vi "Start Power Meter Sweep.vi"(8 "error in (no error)":errorcluster, 10 "Power Meter Sweep (1: Pause)":i32(ring)=1 items=["Run", "Pause"], 11 "VISA resource name":refnum<visa-resource-name>) -> (0 "error out":errorcluster, 3 "VISA resource name out":refnum<visa-resource-name>)   [LabVIEW 2022 SP3, in "Agilent N934X Series.lvlib"]
doc: "Enables or disables power meter sweep state.\n\nNote:\nThis VI is only applicable for N9321C, N9322C, N9323C, N9324C."
uses:
  <instrlib>/Agilent N934X Series/Agilent N934X Series.lvlib
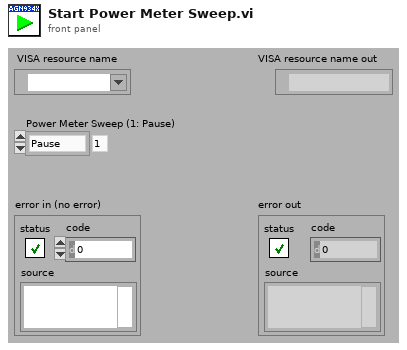
[diagram p1: front panel]
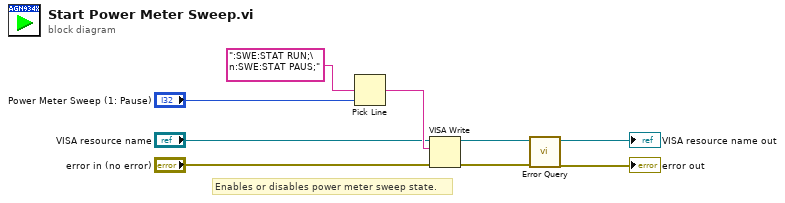
[diagram p0: block diagram]
diagram:
  # "Enables or disables power meter sweep state."
  n1 = Pick Line(multi-line string=":SWE:STAT RUN;\n:SWE:STAT PAUS;", line index="Power Meter Sweep (1: Pause)") -> (output string=w7:string)  [unwired: 1 in]
  n2 = VISA Write(VISA resource name="VISA resource name", write buffer=w7, error in (no error)="error in (no error)") -> (VISA resource name out=w4:refnum<visa-resource-name>, error out=w3:errorcluster)  [unwired: 1 out]
  n3 = call <instrlib>:"Error Query.vi"("error in (no error)"=w3, "VISA resource name"=w4) -> ("error out"=→"error out":errorcluster, "VISA resource name out"=→"VISA resource name out":refnum<visa-resource-name>)  [unwired: 6 in, 2 out]
